vi "Compile.vi"(6 "LocalCompiledDir":path, 7 "DevMode":bool, 8 "error in":errorcluster, 11 "RasPi Compiler in":refnum<class "RasPi Compiler.lvclass">) -> (0 "error out":errorcluster, 3 "RasPi Compiler out":refnum<class "RasPi Compiler.lvclass">)   [LabVIEW 2014, in "RasPi Compiler.lvclass"]
uses:
  RasPi Compiler.lvclass
  RasPi Compiler.lvclass/RasPi Compiler.ctl
  RasPi_Services/MessageBox/MessageBox.lvclass
  VI Interpreter/Classes/VI Interpreter/VI Interpreter.lvclass
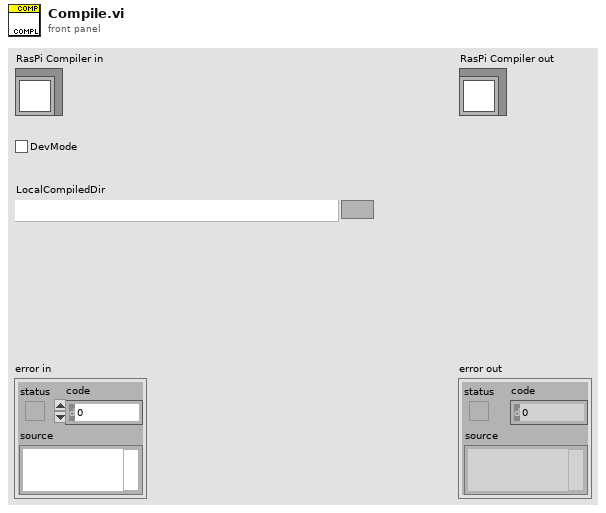
[diagram p1: front panel]
types:
  T1 = typedef "CompileType.ctl" = enum16{"Full GUI", "Console App"}
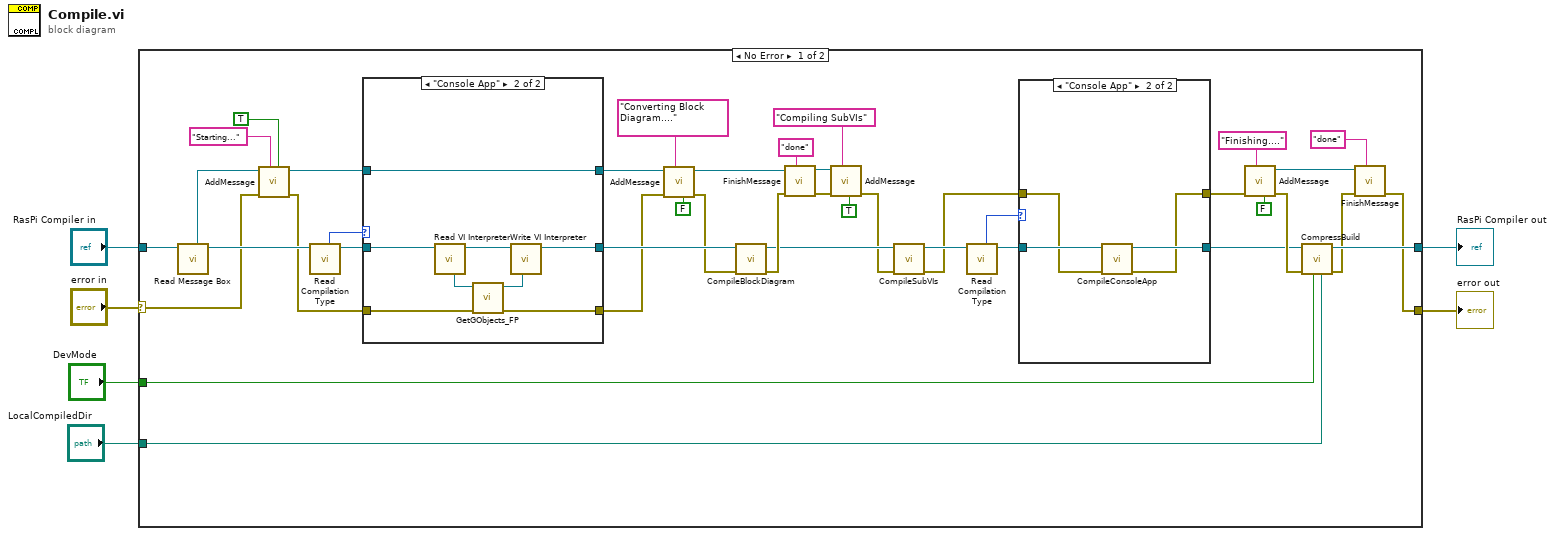
[diagram p0: block diagram]
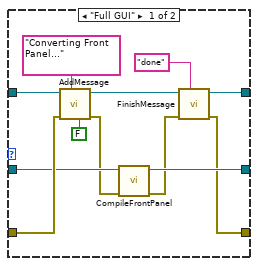
[diagram p3: hidden frame]
diagram:
  n1 = case shown="No Error" "error in" {
    selector: "error in" -> [w38 w75]
    tunnel: [w44 w75] -> w5
    tunnel: [w45 w74] -> w3
    tunnel: "RasPi Compiler in" -> [w43 w74]
    tunnel: "DevMode" -> [w26 _]
    tunnel: "LocalCompiledDir" -> [w25 _]
    frame No Error {
      n2 = call "Read Message Box.vi"("RasPi Compiler in"=w43) -> ("RasPi Compiler out"=w39:refnum<class "RasPi Compiler.lvclass">, "Message Box"=w42:refnum<class "MessageBox.lvclass">)  [unwired: 7 in]
      n3 = call "AddMessage.vi"("add newline"=TRUE, "message"="Starting...", "error in"=w38, "MessageBox in"=w42) -> ("error out"=w37:errorcluster, "MessageBox out"=w36:refnum<class "MessageBox.lvclass">)  [unwired: 4 in]
      n4 = call "Read Compilation Type.vi"("RasPi Compiler in"=w39) -> ("RasPi Compiler out"=w46:refnum<class "RasPi Compiler.lvclass">, "Compilation Type"=w47:T1)  [unwired: 7 in]
      n5 = case shown="\"Console App\"" w47 {
        tunnel: w46 -> [w61 w72]
        tunnel: w37 -> [w62 w69]
        tunnel: [w58 w70] -> w35
        tunnel: [w56 w66] -> w31
        tunnel: w36 -> [w65 w73]
        tunnel: [w55 w73] -> w32
        frame "Full GUI" {
          n6 = call "AddMessage.vi"("add newline"=FALSE, "message"="Converting Front Panel...", "error in"=w62, "MessageBox in"=w65) -> ("error out"=w60:errorcluster, "MessageBox out"=w59:refnum<class "MessageBox.lvclass">)  [unwired: 4 in]
          n7 = call "CompileFrontPanel.vi"("error in"=w60, "RasPi Compiler in"=w61) -> ("error out"=w57:errorcluster, "RasPi Compiler out"=w58:refnum<class "RasPi Compiler.lvclass">)  [unwired: 8 in]
          n8 = call "FinishMessage.vi"("no error"="done", "error in"=w57, "MessageBox in"=w59) -> ("error out"=w56:errorcluster, "MessageBox out"=w55:refnum<class "MessageBox.lvclass">)  [unwired: 5 in]
        }
        frame "Console App" {
          n9 = call "Read VI Interpreter.vi"("RasPi Compiler in"=w72) -> ("RasPi Compiler out"=w71:refnum<class "RasPi Compiler.lvclass">, "VI Interpreter"=w68:refnum<class "VI Interpreter.lvclass">)  [unwired: 7 in]
          n10 = call "GetGObjects_FP.vi"("error in"=w69, "VI Interpreter in"=w68) -> ("error out"=w66:errorcluster, "VI Interpreter out"=w67:refnum<class "VI Interpreter.lvclass">)  [unwired: 8 in]
          n11 = call "Write VI Interpreter.vi"("VI Interpreter"=w67, "RasPi Compiler in"=w71) -> ("RasPi Compiler out"=w70:refnum<class "RasPi Compiler.lvclass">)  [unwired: 7 in]
        }
      }
      n12 = call "AddMessage.vi"("add newline"=FALSE, "message"="Converting Block Diagram....", "error in"=w31, "MessageBox in"=w32) -> ("error out"=w30:errorcluster, "MessageBox out"=w28:refnum<class "MessageBox.lvclass">)  [unwired: 4 in]
      n13 = call "CompileBlockDiagram.vi"("error in"=w30, "RasPi Compiler in"=w35) -> ("error out"=w27:errorcluster, "RasPi Compiler out"=w24:refnum<class "RasPi Compiler.lvclass">)  [unwired: 8 in]
      n14 = call "FinishMessage.vi"("no error"="done", "error in"=w27, "MessageBox in"=w28) -> ("error out"=w20:errorcluster, "MessageBox out"=w22:refnum<class "MessageBox.lvclass">)  [unwired: 5 in]
      n15 = call "AddMessage.vi"("add newline"=TRUE, "message"="Compiling SubVIs", "error in"=w20, "MessageBox in"=w22) -> ("error out"=w18:errorcluster)  [unwired: 4 in, 1 out]
      n16 = call "CompileSubVIs.vi"("error in"=w18, "RasPi Compiler in"=w24) -> ("error out"=w8:errorcluster, "RasPi Compiler out"=w23:refnum<class "RasPi Compiler.lvclass">)  [unwired: 8 in]
      n17 = call "Read Compilation Type.vi"("RasPi Compiler in"=w23) -> ("RasPi Compiler out"=w10:refnum<class "RasPi Compiler.lvclass">, "Compilation Type"=w11:T1)  [unwired: 7 in]
      n18 = case shown="\"Console App\"" w11 {
        tunnel: w10 -> [w49 w53]
        tunnel: [w49 w52] -> w9
        tunnel: w8 -> [w48 w51]
        tunnel: [w48 w50] -> w7
        frame Default {
        }
        frame "Console App" {
          n19 = call "CompileConsoleApp.vi"("error in"=w51, "RasPi Compiler in"=w53) -> ("error out"=w50:errorcluster, "RasPi Compiler out"=w52:refnum<class "RasPi Compiler.lvclass">)  [unwired: 8 in]
        }
      }
      n20 = call "AddMessage.vi"("add newline"=FALSE, "message"="Finishing....", "error in"=w7) -> ("error out"=w15:errorcluster, "MessageBox out"=w14:refnum<class "MessageBox.lvclass">)  [unwired: 5 in]
      n21 = call "CompressBuild.vi"("LocalCompiledDir"=w25, "DevMode"=w26, "error in"=w15, "RasPi Compiler in"=w9) -> ("error out"=w13:errorcluster, "RasPi Compiler out"=w45:refnum<class "RasPi Compiler.lvclass">)  [unwired: 6 in]
      n22 = call "FinishMessage.vi"("no error"="done", "error in"=w13, "MessageBox in"=w14) -> ("error out"=w44:errorcluster)  [unwired: 5 in, 1 out]
    }
    frame Error {
    }
  }
  "error out" <- w5
  "RasPi Compiler out" <- w3
